vi "Decode Fixed Header.vi"(8 "error in (no error)":errorcluster, 11 "String":string) -> (0 "error out":errorcluster, 3 "Fixed Header":T1)   [LabVIEW 2023, in "WebSocket.lvclass"]
uses:
  WebSocket.lvclass
  private/Fixed Header.ctl
  private/OpCode.ctl
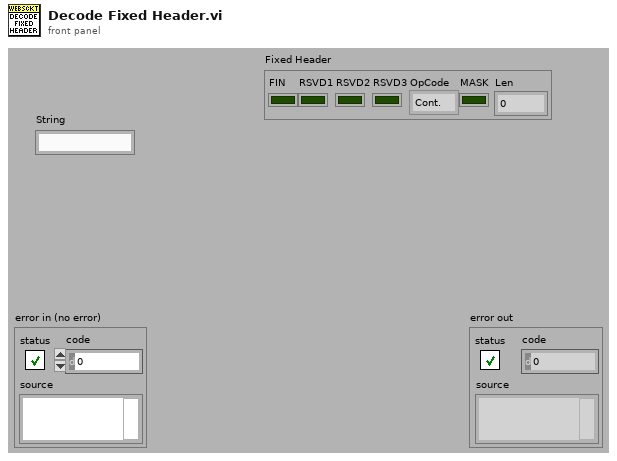
[diagram p1: front panel]
types:
  T1 = typedef "WebSocket.lvclass/Fixed Header.ctl" = cluster{"FIN":bool, "RSVD1":bool, "RSVD2":bool, "RSVD3":bool, "OpCode":T2, "MASK":bool, "Len":u8}
  T2 = typedef "WebSocket.lvclass/OpCode.ctl" = enum16{"Cont.", "Text", "Binary", "NonCtl3", "NonCtl4", "NonCtl5", "NonCtl6", "NonCtl7", "Close", "Ping", "Pong", "Rsvd11", "Rsvd12", "Rsvd13", "Rsvd14", "Rsvd15"}
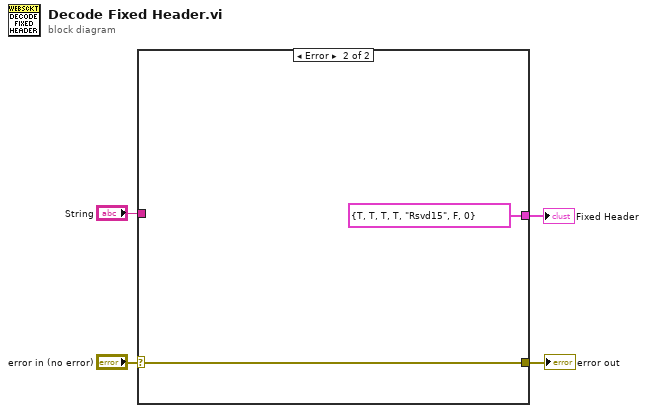
[diagram p0: block diagram]
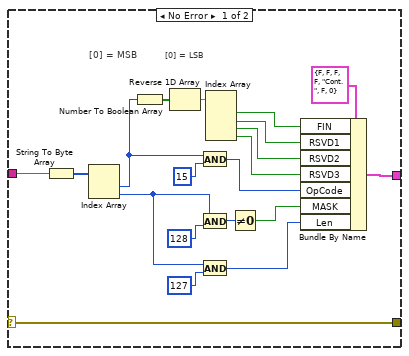
[diagram p2: hidden frame]
diagram:
  n1 = case shown="Error" "error in (no error)" {
    selector: "error in (no error)" -> [w5 w26]
    tunnel: "String" -> [w24 _]
    tunnel: [w20 T1 {"FIN"=TRUE, "RSVD1"=TRUE, "RSVD2"=TRUE, "RSVD3"=TRUE, "OpCode"=enum."Rsvd15", "MASK"=FALSE, "Len"=0} ("Fixed Header")] -> w3
    tunnel: [w5 w26] -> w1
    frame No Error {
      # "[0] = LSB"
      # "[0] = MSB"
      n2 = String To Byte Array(string=w24) -> (unsigned byte array=w23:u8[])
      n3 = Index Array(array=w23) -> (element #1=w15:u8, element #2=w8:u8)  [unwired: 2 in]
      n4 = Number To Boolean Array(number=w15) -> (Boolean array=w22:bool[])
      n5 = Reverse 1D Array(array=w22) -> (reversed array=w6:bool[])
      n6 = And(x=w15, y=u8 15) -> (x .and. y?=w13:u8)
      n7 = And(x=w8, y=u8 128) -> (x .and. y?=w11:u8)
      n8 = And(x=w8, y=u8 127) -> (x .and. y?=w7:u8)
      n9 = Index Array(array=w6) -> (element #1=w19:bool, element #2=w18:bool, element #3=w17:bool, element #4=w16:bool)  [unwired: 4 in]
      n10 = Not Equal To 0?(x=w11) -> (x != 0?=w10:bool)
      n11 = Bundle By Name(cluster=T1 {"FIN"=FALSE, "RSVD1"=FALSE, "RSVD2"=FALSE, "RSVD3"=FALSE, "OpCode"=enum."Cont.", "MASK"=FALSE, "Len"=0} ("Fixed Header"), "FIN"=w19, "RSVD1"=w18, "RSVD2"=w17, "RSVD3"=w16, "OpCode"=w13, "MASK"=w10, "Len"=w7) -> (w20:T1)
    }
    frame Error {
    }
  }
  "error out" <- w1
  "Fixed Header" <- w3
